vi "Receive Boolean.vi"(8 "error in (no error)":errorcluster, 10 "Broadcast Boolean Msg":refnum<class "Broadcast Boolean Msg.lvclass">, 11 "TopLevelApplication In":refnum<class "TopLevelApplication.lvclass">) -> (0 "error out":errorcluster, 3 "TopLevelApplication Out":refnum<class "TopLevelApplication.lvclass">)   [LabVIEW 2015, in "TopLevelApplication.lvlib" / "TopLevelApplication.lvclass"]
uses:
  TopLevelApplication.lvclass
  IViewable/IViewable Messages/Broadcast Boolean Msg/Broadcast Boolean Msg.lvclass
  IViewable/IViewable Messages/Broadcast Boolean Msg/Broadcast Boolean Msg.lvclass/Broadcast Boolean Msg.ctl
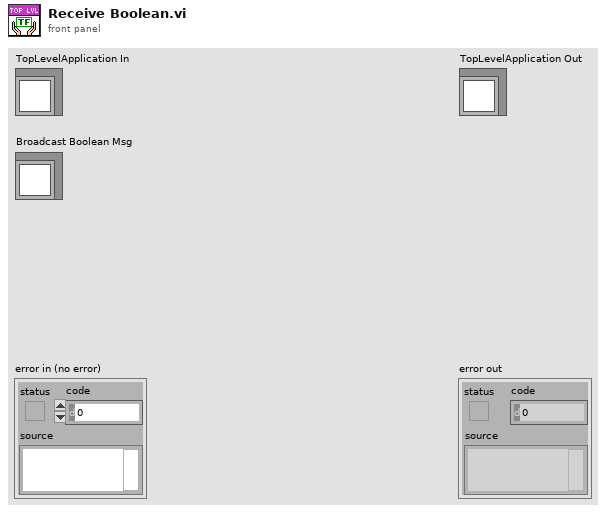
[diagram p1: front panel]
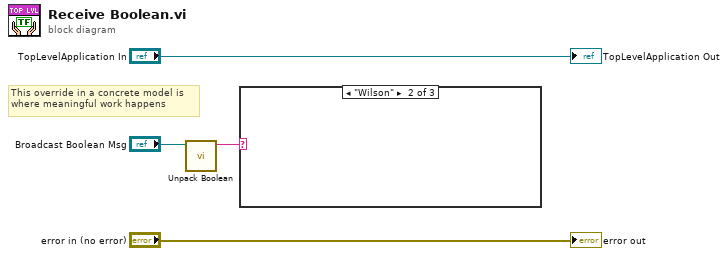
[diagram p0: block diagram]
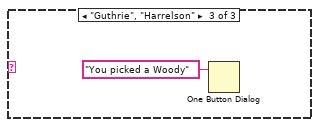
[diagram p3: hidden frame]
diagram:
  # "This override in a concrete model is\nwhere meaningful work happens"
  n1 = call "Unpack Boolean.vi"("Broadcast Boolean Msg In"="Broadcast Boolean Msg") -> ("Control Label"=w1:string)  [unwired: 9 in, 1 out]
  n2 = case shown="\"Wilson\"" w1 {
    frame Default {
    }
    frame "Wilson" {
    }
    frame "Guthrie", "Harrelson" {
      n3 = One Button Dialog(message="You picked a Woody") -> ()  [unwired: 1 in, 1 out]
    }
  }
  "error out" <- "error in (no error)"
  "TopLevelApplication Out" <- "TopLevelApplication In"
